vi "Experiment_Init.vi"(0 "object in":refnum<class "Experiment.lvclass">, 2 "Path":path, 5 "error in (no error)":errorcluster) -> (14 "object out":refnum<class "Experiment.lvclass">, 16 "file or folder exists?":bool, 19 "error out":errorcluster)   [LabVIEW 2021, in "Experiment.lvclass"]
uses:
  Experiment.lvclass
  Experiment.lvclass/Experiment.ctl
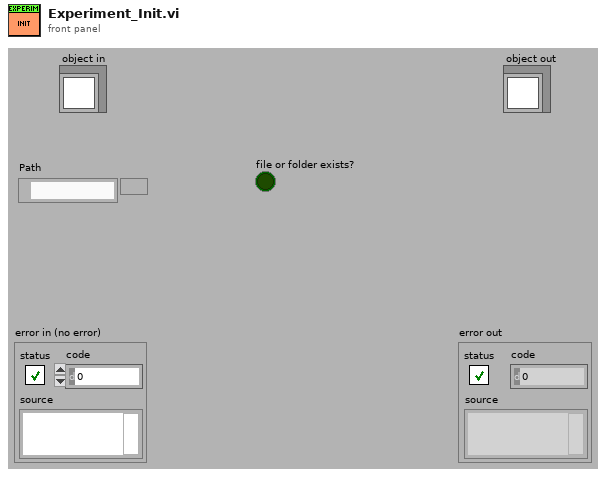
[diagram p1: front panel]
types:
  T1 = enum16{"open", "open or create", "create or replace", "create", "open (read-only)"}
  T2 = cluster{"Message":string, "Message Data":variant, "Wait Command":bool}
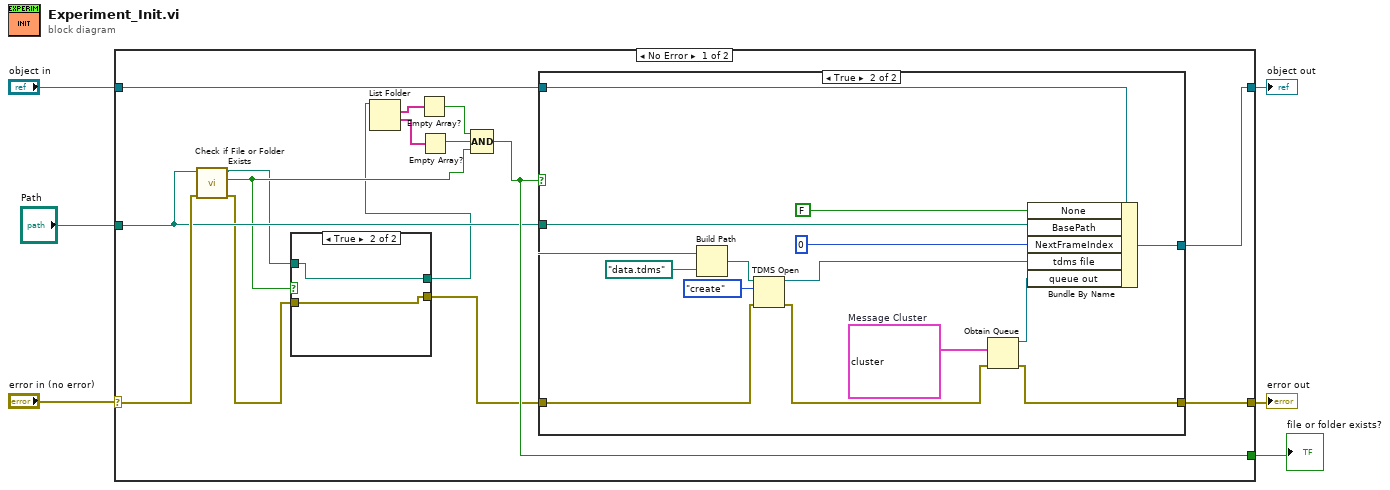
[diagram p0: block diagram]
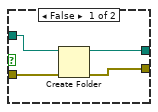
[diagram p2: hidden frame]
diagram:
  n1 = case shown="No Error" "error in (no error)" {
    selector: "error in (no error)" -> [w18 w44]
    tunnel: "object in" -> [w21 w45]
    tunnel: [w20 w45] -> w5
    tunnel: [w19 w44] -> w3
    tunnel: "Path" -> [w12 _]
    tunnel: [w13 _] -> w1
    frame No Error {
      n2 = call <vilib>:"Check if File or Folder Exists.vi"("error in (no error)"=w18, "path"=w12) -> ("error out"=w8:errorcluster, "file or folder exists?"=w11:bool, "dup path"=w10:path)  [unwired: 7 in]
      n3 = case shown="True" w11 {
        tunnel: w10 -> [w25 w27]
        tunnel: [w24 w27] -> w9
        tunnel: w8 -> [w23 w26]
        tunnel: [w22 w26] -> w7
        frame False {
          n4 = Create Folder(path (use dialog)=w25, error in=w23) -> (created path=w24:path, error out=w22:errorcluster)  [unwired: 1 in, 1 out]
        }
        frame True {
        }
      }
      n5 = List Folder(path=w9) -> (filenames=w16:string[], folder names=w17:string[])  [unwired: 3 in, 2 out]
      n6 = Empty Array?(array=w16) -> (empty?=w14:bool)
      n7 = Empty Array?(array=w17) -> (empty?=w15:bool)
      n8 = Compound Arithmetic op=AND(w14, w15, w11) -> (w13:bool)
      n9 = case shown="True" w13 {
        tunnel: w21 -> [w29 w43]
        tunnel: [w29 w42] -> w20
        tunnel: [w28 w33] -> w19
        tunnel: w12 -> [_ w32]
        tunnel: w7 -> [w28 w31]
        frame False {
        }
        frame True {
          w35 = T2 {"Message"="", "Message Data"=variant, "Wait Command"=TRUE}  # Message Cluster
          n10 = Build Path(base path=w32, name or relative path=path "data.tdms") -> (appended path=w39:path)
          n11 = TDMS Open(8:w31, 10:T1."create" ("operation (0:open)"), 11:w39) -> (0:w34:errorcluster, 3:w36:refnum<k34>)  [unwired: 4 in]
          n12 = Obtain Queue(element data type=w35, error in (no error)=w34) -> (queue out=w30:refnum<queue>, error out=w33:errorcluster)  [unwired: 3 in, 1 out]
          n13 = Bundle By Name(cluster=w43, "None"=FALSE, "BasePath"=w32, "NextFrameIndex"=u16 0, "tdms file"=w36, "queue out"=w30) -> (w42:refnum<class "Experiment.lvclass">)
        }
      }
    }
    frame Error {
    }
  }
  "object out" <- w5
  "error out" <- w3
  "file or folder exists?" <- w1
